vi "Lookup Node.vi"(7 "Start (Root)":refnum<class "Config Element.lvclass">, 8 "error in (no error)":errorcluster, 10 "Node Name":string, 11 "VolatusConfig in":refnum<class "VolatusConfig.lvclass">) -> (0 "error out":errorcluster, 2 "Node":refnum<class "Node.lvclass">, 3 "VolatusConfig out":refnum<class "VolatusConfig.lvclass">)   [LabVIEW 2020, in "VolatusConfig.lvlib" / "VolatusConfig.lvclass"]
uses:
  VolatusConfig.lvclass
  lv-cdm/CDM-Config/Config Element/Config Element.lvclass
  Node/Node.lvclass
  Meta Name.ctl
  Meta Type.ctl
  VolatusConfig.lvclass/VolatusConfig.ctl
  VolatusConfig.lvlib
  lv-cdm/CDM-Config/Config Filter/Config Lookup.lvclass
  lv-cdm/CDM-Config/Config Manager/Config Manager.lvclass
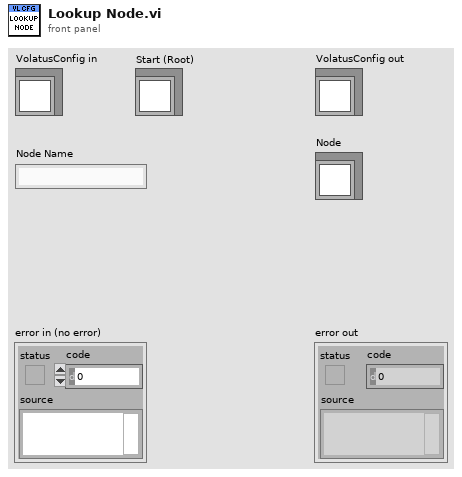
[diagram p1: front panel]
types:
  T1 = typedef "VolatusConfig.lvlib/Meta Type.ctl" = enum16{"UNKNOWN", "VL_System", "VL_Cluster", "VL_Node", "VL_Task", "VL_Group", "VL_Channel", "VL_Task_List", "VL_Scaling", "VL_Sensor", "VL_Sensor_List", "VL_Scale"}
  T2 = typedef "VolatusConfig.lvlib/Meta Name.ctl" = enum16{"VL_Type", "VL_Node_IP", "VL_Node_Type", "VL_Task_Type", "VL_Group_Type", "VL_Channel_Type", "VL_Channel_DataType", "VL_Config_Version", "VL_Overlay_Type"}
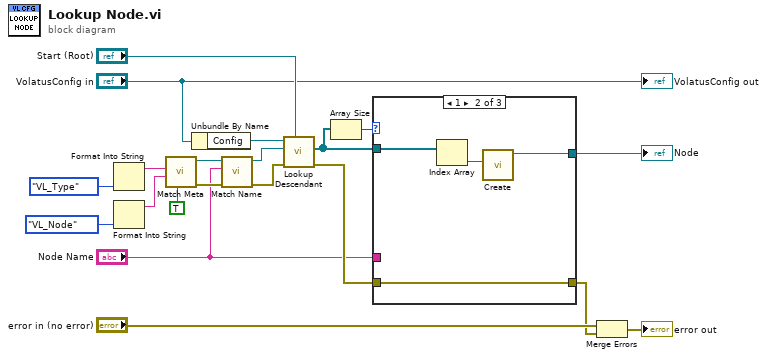
[diagram p0: block diagram]
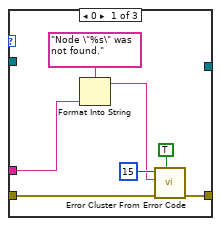
[diagram p2: hidden frame]
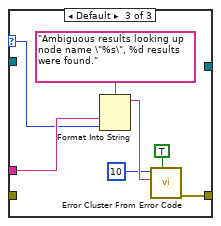
[diagram p3: hidden frame]
diagram:
  n1 = Format Into String(Meta_Name."VL_Type" ("Meta Name")) -> (resulting string=w17:string)  [unwired: 3 in, 1 out]
  n2 = Format Into String(Meta_Type."VL_Node" ("input 1")) -> (resulting string=w16:string)  [unwired: 3 in, 1 out]
  n3 = call "Match Meta.vi"("Exact Value (F)"=TRUE, "Value (Any)"=w16, "Name"=w17) -> ("error out"=w20:errorcluster, "Config Lookup out"=w5:refnum<class "Config Lookup.lvclass">)  [unwired: 7 in]
  n4 = Unbundle By Name("VolatusConfig in") -> ("Config"=w12:refnum<class "Config Manager.lvclass">)
  n5 = call "Match Name.vi"("error in (no error)"=w20, "Name"="Node Name", "Config Lookup (New)"=w5) -> ("error out"=w2:errorcluster, "Config Lookup out"=w3:refnum<class "Config Lookup.lvclass">)  [unwired: 7 in]
  n6 = call "Lookup Descendant.vi"("Start (Root)"="Start (Root)", "error in (no error)"=w2, "Lookup"=w3, "Config Manager in"=w12) -> ("error out"=w7:errorcluster, "Descendants"=w9:refnum<class "Config Element.lvclass">[])  [unwired: 5 in, 1 out]
  n7 = Array Size(array=w9) -> (size(s)=w10:i32)
  n8 = case shown="1" w10 {
    selector: w10 -> [_ _ w32]
    tunnel: w9 -> [_ w31 _]
    tunnel: [_ w28 _] -> w8
    tunnel: w7 -> [w24 w29 _]
    tunnel: "Node Name" -> [w21 _ w33]
    tunnel: [w23 w29 w36] -> w6
    frame 0 {
      n9 = Format Into String(format string="Node \"%s\" was not found.", w21) -> (resulting string=w22:string)  [unwired: 2 in, 1 out]
      n10 = call <vilib>:"Error Cluster From Error Code.vi"("show call chain? (False)"=TRUE, "error in (no error)"=w24, "error message (\"\")"=w22, "error code (0)"=15) -> ("error out"=w23:errorcluster)  [unwired: 5 in]
    }
    frame 1 {
      n11 = Index Array(array=w31) -> (element=w30:refnum<class "Config Element.lvclass">)  [unwired: 1 in]
      n12 = call "Create.vi"("Element"=w30) -> ("Node out"=w28:refnum<class "Node.lvclass">)  [unwired: 9 in, 1 out]
    }
    frame Default {
      n13 = Format Into String(format string="Ambiguous results looking up node name \"%s\", %d results were found.", w33, w32) -> (resulting string=w35:string)  [unwired: 2 in, 1 out]
      n14 = call <vilib>:"Error Cluster From Error Code.vi"("show call chain? (False)"=TRUE, "error message (\"\")"=w35, "error code (0)"=10) -> ("error out"=w36:errorcluster)  [unwired: 6 in]
    }
  }
  "Node" <- w8
  n15 = Merge Errors("error in (no error)", w6) -> (→"error out":errorcluster)
  "VolatusConfig out" <- "VolatusConfig in"
